vi "quaternion_normalize.vi"(11 "q1 * q2":dbl[](array[numeric])) -> (3 "normalized vector":dbl[](array[numeric]))   [LabVIEW 2012]
uses:
  norm_vec.vi
panel:
  # "As well as normalizing the magnitude, we flip the sign to keep W (the real part) positive.   This canonicalizes the quaternion and avoids singularities in the axis/angle conversion near 360 degrees."
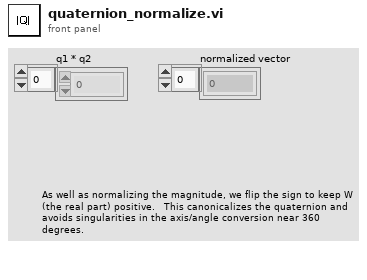
[diagram p1: front panel]
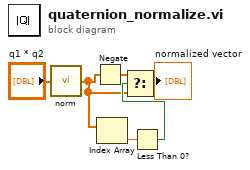
[diagram p0: block diagram]
diagram:
  n1 = call-poly "norm.vi"("vector"="q1 * q2") -> ("normalized vector"=w4:dbl[])  [unwired: 3 in, 1 out]
  n2 = Negate(x=w4) -> (-x=w3:dbl[])
  n3 = Index Array(array=w4) -> (element=w2:dbl)  [unwired: 1 in]
  n4 = Less Than 0?(x=w2) -> (x < 0?=w5:bool)
  n5 = Select(t=w3, s=w5, f=w4) -> (s? t:f=→"normalized vector":dbl[])
